vi "HFRR ADV v027 new software.vi"() -> ()   [LabVIEW 2025] (continued)
                      n2898 = Fract/Exp String To Number(string=w3966) -> (number=→"MWSD 2":dbl)  [unwired: 3 in, 1 out]
                    }
                    frame 11 {
                      n2899 = Fract/Exp String To Number(string=w3968) -> (number=→"AVP 2":dbl)  [unwired: 3 in, 1 out]
                    }
                    frame 12 {
                      n2900 = Fract/Exp String To Number(string=w3970) -> (number=→"HCF 2":dbl)  [unwired: 3 in, 1 out]
                    }
                    frame 13 {
                      n2901 = Fract/Exp String To Number(string=w3972) -> (number=→"WS1.4 2":dbl)  [unwired: 3 in, 1 out]
                    }
                    frame 14, Default {
                    }
                  }
                }
              }
              frame #2 {
              }
            }
            n2902 = local write "OK Button 16"(FALSE ("OK Button 13")) -> ()
          }
        }
        n2903 = Index Array(array=w3617, index="Select Printer 3") -> (element=w3619:string)
        "Selected Printer" <- w3619
        n2904 = case shown="True" w3614 {
          frame False {
          }
          frame True {
            n2905 = flat-sequence {
              frame #0 {
              }
              frame #1 {
                n2906 = Wait (ms)(milliseconds to wait=u32 100) -> ()  [unwired: 1 out]
              }
              frame #2 {
                n2907 = local write "OK Button 16"(FALSE ("Print 3")) -> ()
              }
            }
          }
        }
        n2908 = case shown="True" "Print" {
          tunnel: w3619 -> [_ w3911]
          frame False {
          }
          frame True {
            (unwired) i16 6 ("width (-)")
            (unwired) "TESTED BY : "
            (unwired) "TESTED DATE :"
            (unwired) "SAMPLE ID : "
            (unwired) "SAMPLE DESIGN : "
            w3869 = "\r"
            w3886 = "\r"
            # "add image"
            n2909 = local read "Sample ID"() -> (w3859:string)
            n2910 = local read "Tested by"() -> (w3862:string)
            n2911 = local read "String 34"() -> (w3849:string)
            n2912 = local read "String 45"() -> (w3829:string)
            n2913 = local read "String 35"() -> (w3844:string)
            n2914 = local read "String 37"() -> (w3842:string)
            n2915 = local read "String 32"() -> (w3864:string)
            n2916 = local read "String 36"() -> (w3839:string)
            n2917 = local read "String 31"() -> (w3863:string)
            n2918 = local read "Test Date"() -> (w3860:string)
            n2919 = local read "String 33"() -> (w3865:string)
            n2920 = local read "String 38"() -> (w3835:string)
            n2921 = local read "String 39"() -> (w3832:string)
            n2922 = local write "Print"(FALSE ("Print FF")) -> ()
            n2923 = local read "S 39"() -> (w3847:string)
            n2924 = local read "S 38"() -> (w3854:string)
            n2925 = local read "Temperature before test 2"() -> (w3885:dbl)
            n2926 = local read "Temperature after test 2"() -> (w3875:dbl)
            n2927 = local read "Humidity before test 2"() -> (w3900:dbl)
            n2928 = local read "Humidity after test 2"() -> (w3884:dbl)
            n2929 = local read "MWSD 2"() -> (w3889:dbl)
            n2930 = local read "WS1.4 2"() -> (w3867:dbl)
            n2931 = Concatenate Strings("2)" ("string"), w3849) -> (w3850:string)
            n2932 = Concatenate Strings("3)" ("string"), w3847) -> (w3848:string)
            n2933 = Concatenate Strings("1)" ("string"), w3854) -> (w3853:string)
            n2934 = Concatenate Strings("4)" ("string"), w3844) -> (w3845:string)
            n2935 = Concatenate Strings("5)" ("string"), w3842) -> (w3841:string)
            n2936 = Concatenate Strings("6)" ("string"), w3839) -> (w3838:string)
            n2937 = Concatenate Strings("7)" ("string"), w3835) -> (w3836:string)
            n2938 = Concatenate Strings("8)" ("string"), w3832) -> (w3833:string)
            n2939 = local read "HCF 2"() -> (w3871:dbl)
            n2940 = local read "AVP 2"() -> (w3888:dbl)
            n2941 = local read "s.NO"() -> (w3830:string)
            n2942 = call <vilib>:"New Report.vi"("report type"=enum16{"Standard Report", "HTML"}."Standard Report") -> ("report out"=w3909:refnum<class "NI_report.lvclass">, "error out"=w3908:errorcluster)  [unwired: 13 in]
            n2943 = local read "TITTLE"() -> (w3861:string)
            n2944 = Concatenate Strings(w3886, w3829, w3830, w3886, w3864, w3859, w3886, w3863, w3860, w3886, w3865, w3862, w3886) -> (w3879:string)
            "test by" <- w3879
            n2945 = Number To Fractional String(number=w3885, width (-)=i16 6, precision (6)=i16 2) -> (F-format string=w3874:string)  [unwired: 1 in]
            n2946 = Number To Fractional String(number=w3884, width (-)=i16 6, precision (6)=i16 2) -> (F-format string=w3887:string)  [unwired: 1 in]
            n2947 = Number To Fractional String(number=w3900, width (-)=i16 6, precision (6)=i16 2) -> (F-format string=w3905:string)  [unwired: 1 in]
            n2948 = Number To Fractional String(number=w3889, width (-)=i16 6, precision (6)=i16 2) -> (F-format string=w3891:string)  [unwired: 1 in]
            n2949 = Number To Fractional String(number=w3875, width (-)=i16 6, precision (6)=i16 2) -> (F-format string=w3876:string)  [unwired: 1 in]
            n2950 = Number To Fractional String(number=w3888, width (-)=i16 6, precision (6)=i16 2) -> (F-format string=w3890:string)  [unwired: 1 in]
            n2951 = Number To Fractional String(number=w3871, width (-)=i16 6, precision (6)=i16 2) -> (F-format string=w3870:string)  [unwired: 1 in]
            n2952 = Number To Fractional String(number=w3867, precision (6)=i16 2) -> (F-format string=w3866:string)  [unwired: 2 in]
            n2953 = call-dynamic "Set Report Header Text.vi"("report in"=w3909, "center header text"=w3861, "error in (no error)"=w3908) -> ("report out"=w3880:refnum<class "NI_report.lvclass">, "error out"=w3881:errorcluster)  [unwired: 11 in]
            n2954 = Concatenate Strings(w3869, w3853, w3905, w3869, w3850, w3874, w3869, w3848, w3887, w3869, w3845, w3876, w3869, w3841, w3891, w3869, w3838, w3890, w3869, w3836, w3870, w3869, w3833, w3866) -> (w3857:string)
            "export 2" <- w3857
            n2955 = call-poly <vilib>:"Append Report Text.vi"("report in"=w3880, "text"=w3879, "error in (no error)"=w3881) -> ("report out"=w3883:refnum<class "NI_report.lvclass">, "error out"=w3882:errorcluster)  [unwired: 9 in, 2 out]
            n2956 = local read "test by"() -> (w3856:string)
            n2957 = local read "TITTLE"() -> (w3858:string)
            n2958 = call-poly <vilib>:"Append Report Text.vi"("report in"=w3883, "error in (no error)"=w3882) -> ("report out"=w3904:refnum<class "NI_report.lvclass">, "error out"=w3902:errorcluster)  [unwired: 10 in, 2 out]
            n2959 = Concatenate Strings(w3858, w3857, w3856) -> (→"output":string)
            n2960 = call-poly <vilib>:"Append Report Text.vi"("report in"=w3904, "text"=w3857, "error in (no error)"=w3902) -> ("report out"=w3903:refnum<class "NI_report.lvclass">, "error out"=w3901:errorcluster)  [unwired: 9 in, 2 out]
            n2961 = call-dynamic "Print Report.vi"("report in"=w3903, "printer name (default)"=w3911, "error in (no error)"=w3901) -> ("report out"=w3913:refnum<class "NI_report.lvclass">, "error out"=w3914:errorcluster)  [unwired: 11 in]
            n2962 = call-dynamic "Dispose Report.vi"("report in"=w3913, "error in (no error)"=w3914) -> ()  [unwired: 13 in, 1 out]
          }
        }
        n2963 = case shown="True" "Print 2" {
          frame False {
          }
          frame True {
            n2964 = flat-sequence {
              frame #0 {
                n2965 = local read "s.NO"() -> (→"s.NO 2":string)
                n2966 = Wait (ms)(milliseconds to wait=u32 20) -> ()  [unwired: 1 out]
                n2967 = local read "Sample ID  3"() -> (→"Sample ID  6":string)
                n2968 = local read "Sample ID  4"() -> (→"Sample ID  7":string)
                n2969 = local read "Sample ID"() -> (→"Sample ID  2":string)
                n2970 = local read "Tested by"() -> (→"Tested by 2":string)
                n2971 = local read "Test Date"() -> (→"Test Date 2":string)
                n2972 = local read "Humidity after test 3"() -> (→"Humidity after test 4":dbl)
                n2973 = local read "Ref A Test Date :"() -> (→"TITTLE 4":string)
                n2974 = local read "Temperature before test 3"() -> (w3736:dbl)
                n2975 = local read "Temperature before test 3"() -> (→"Temperature after test 5":dbl)
                n2976 = local read "Temperature after test 3"() -> (→"Temperature after test 4":dbl)
                n2977 = local read "Humidity before test 3"() -> (→"Humidity before test 4":dbl)
                n2978 = local write "Temperature before test 3"(w3736) -> ()
                n2979 = local read "image data"() -> (w3727:T16)
                n2980 = String To Path(string="C:\\LAB-IQ\\im\\Temp_resized.jpg") -> (path=w3728:path)
                "path 2" <- w3728
                n2981 = call <vilib>:"Write JPEG File.vi"("image data"=w3727, "path to JPEG file"=w3728) -> ()  [unwired: 8 in, 2 out]
                "Ref A Test Date :" <- "Ref A Test Date :"
                "Ref B Test Date :" <- "Ref B Test Date :"
                "Ref B Scar Value :" <- "Ref B Scar Value :"
                "Ref A Scar Value :" <- "Ref A Scar Value :"
              }
              frame #1 {
                (unwired) HTML_Report_Image_Alignment."MIDDLE" ("alignment (default)")
                w3764 = u16 0 items=["portrait", "landscape"] ("orientation (portrait)")
                (unwired) HTML_Report_Image_Alignment."ABSMIDDLE" ("alignment (default)")
                (unwired) "TESTED BY : "
                (unwired) "TESTED DATE :"
                (unwired) "SAMPLE ID : "
                (unwired) "SAMPLE DESIGN : "
                w3797 = "\r"
                # "add image"
                n2982 = Wait (ms)(milliseconds to wait=u32 20) -> ()  [unwired: 1 out]
                n2983 = local read "Sample ID  2"() -> (w3790:string)
                n2984 = local read "Wear Scar X"() -> (w3762:dbl)
                "Length ( microns ) 2" <- w3762
                n2985 = local read "Wear Scar Y"() -> (w3761:dbl)
                "Wear Scar Y ( microns ) :" <- w3761
                n2986 = local read "Test Date 2"() -> (w3791:string)
                n2987 = local read "Tested by 2"() -> (w3792:string)
                n2988 = local read "String 46"() -> (w3788:string)
                n2989 = local read "String 48"() -> (w3794:string)
                n2990 = local read "String 47"() -> (w3793:string)
                n2991 = local read "String 49"() -> (w3795:string)
                n2992 = local read "String 10"() -> (w3748:string)
                n2993 = local read "s.NO 2"() -> (w3789:string)
                n2994 = Add(x=w3762, y=w3761) -> (x+y=w3760:dbl)
                n2995 = call <vilib>:"New Report.vi"("report type"=enum16{"Standard Report", "HTML"}."HTML") -> ("report out"=w3768:refnum<class "NI_report.lvclass">, "error out"=w3766:errorcluster)  [unwired: 13 in]
                n2996 = Concatenate Strings(w3797, w3788, w3789, w3797, w3794, w3790, w3797, w3793, w3791, w3797, w3795, w3792, w3797) -> (→"test by 2":string)
                n2997 = Concatenate Strings("C:\\LAB-IQ\\Data\\" ("string"), w3748, ".jpg" ("string")) -> ()  [unwired: 1 out]
                n2998 = Divide(x=w3760, y=2.0) -> (x/y=→"Mean Wear ( microns) :":dbl)
                n2999 = call-dynamic "Set Report Orientation.vi"("report in"=w3768, "orientation (portrait)"=w3764, "error in (no error)"=w3766) -> ("report out"=w3767:refnum<class "NI_report.lvclass">, "error out"=w3765:errorcluster)  [unwired: 11 in]
                n3000 = for {
                  N: 5 -> [_]
                  tunnel: w3767 -> [w3818]
                  tunnel: [w3817] -> w3746
                  tunnel: w3765 -> [w3816]
                  tunnel: [w3815] -> w3745
                  n3001 = call-dynamic "Set Report Tab Width.vi"("report in"=w3818, "error in (no error)"=w3816) -> ("report out"=w3817:refnum<class "NI_report.lvclass">, "error out"=w3815:errorcluster)  [unwired: 12 in]
                }
                n3002 = local read "TITTLE"() -> (w3763:string)
                n3003 = call-dynamic "Set Report Header Text.vi"("report in"=w3746, "center header text"=w3763, "error in (no error)"=w3745) -> ("report out"=w3784:refnum<class "NI_report.lvclass">, "error out"=w3783:errorcluster)  [unwired: 11 in]
                n3004 = for {
                  N: 1 -> [_]
                  tunnel: [w3822] -> w3770
                  tunnel: [w3821] -> w3769
                  tunnel: w3784 -> [w3820]
                  tunnel: w3783 -> [w3819]
                  n3005 = call-dynamic "New Report Line.vi"("report in"=w3820, "error in (no error)"=w3819) -> ("report out"=w3822:refnum<class "NI_report.lvclass">, "error out"=w3821:errorcluster)  [unwired: 12 in]
                }
                n3006 = for {
                  N: 2 -> [_]
                  tunnel: [w3814] -> w3776
                  tunnel: [w3813] -> w3775
                  tunnel: w3770 -> [w3812]
                  tunnel: w3769 -> [w3811]
                  n3007 = call-dynamic "New Report Line.vi"("report in"=w3812, "error in (no error)"=w3811) -> ("report out"=w3814:refnum<class "NI_report.lvclass">, "error out"=w3813:errorcluster)  [unwired: 12 in]
                }
                n3008 = for {
                  N: 25 -> [_]
                  tunnel: w3776 -> [w3810]
                  tunnel: w3775 -> [w3808]
                  tunnel: [w3809] -> w3779
                  tunnel: [w3807] -> w3778
                  n3009 = call-dynamic "Set Report Tab Width.vi"("report in"=w3810, "error in (no error)"=w3808) -> ("report out"=w3809:refnum<class "NI_report.lvclass">, "error out"=w3807:errorcluster)  [unwired: 12 in]
                }
                n3010 = control-ref of="Tab Control 9"() -> (w3774:refnum<vi>)
                n3011 = call-dynamic "Append Control Image to Report.vi"("report in"=w3779, "alignment (default)"=HTML_Report_Image_Alignment."ABSMIDDLE", "ctrl reference"=w3774, "error in (no error)"=w3778) -> ("report out"=w3773:refnum<class "NI_report.lvclass">, "error out"=w3772:errorcluster)  [unwired: 8 in, 2 out]
                n3012 = for {
                  N: 3 -> [_]
                  tunnel: [w3806] -> w3757
                  tunnel: [w3805] -> w3756
                  tunnel: w3773 -> [w3804]
                  tunnel: w3772 -> [w3803]
                  n3013 = call-dynamic "New Report Line.vi"("report in"=w3804, "error in (no error)"=w3803) -> ("report out"=w3806:refnum<class "NI_report.lvclass">, "error out"=w3805:errorcluster)  [unwired: 12 in]
                }
                n3014 = for {
                  N: 100 -> [_]
                  tunnel: w3757 -> [w3802]
                  tunnel: w3756 -> [w3800]
                  tunnel: [w3801] -> w3753
                  tunnel: [w3799] -> w3751
                  n3015 = call-dynamic "Set Report Tab Width.vi"("report in"=w3802, "error in (no error)"=w3800) -> ("report out"=w3801:refnum<class "NI_report.lvclass">, "error out"=w3799:errorcluster)  [unwired: 12 in]
                }
                n3016 = String To Path(string="C:\\LAB-IQ\\im\\Temp_resized.jpg") -> (path=w3743:path)
                n3017 = call-poly <vilib>:"Append Image to Report.vi"("report in"=w3753, "path or URL of image"=w3743, "error in (no error)"=w3751) -> ("report out"=w3752:refnum<class "NI_report.lvclass">, "error out"=w3750:errorcluster)  [unwired: 9 in, 2 out]
                n3018 = call-poly <vilib>:"Open HTML Report in Browser.vi"("report in"=w3752, "error in (no error)"=w3750) -> ("report out"=w3787:refnum<class "NI_report.lvclass">, "error out"=w3786:errorcluster)  [unwired: 11 in, 1 out]
                n3019 = call-dynamic "Dispose Report.vi"("report in"=w3787, "error in (no error)"=w3786) -> ()  [unwired: 13 in, 1 out]
              }
              frame #2 {
              }
              frame #3 {
                n3020 = disable-structure shown="Disabled" {
                  frame Disabled {
                    n3021 = local read "String 10"() -> (w3827:string)
                    n3022 = Concatenate Strings("C:\\LAB-IQ-NXT\\Data\\" ("string"), w3827, ".jpg" ("string")) -> (w3825:string)
                    n3023 = String To Path(string=w3825) -> (path=w3824:path)
                    n3024 = Delete(path (use dialog)=w3824) -> ()  [unwired: 4 in, 3 out]
                  }
                  frame Enabled {
                  }
                }
                n3025 = local write "Print 2"(FALSE ("Print")) -> ()
              }
            }
          }
        }
      }
    }
    n3026 = Wait (ms)(milliseconds to wait=u32 50) -> ()  [unwired: 1 out]
    n3027 = Wait (ms)(milliseconds to wait=u32 50) -> ()  [unwired: 1 out]
    n3028 = local read "Quit"() -> (w2172:bool)
  }
  n3029 = VISA Close(VISA resource name=w41, error in (no error)=w40) -> ()  [unwired: 1 out]
  n3030 = while {
    tunnel: [w3990] -> w49
    shift-right: [w3983] -> _
    shift-left: 0.0 -> [w3986]
    shift-right: [w3982] -> _
    shift-left: 0.0 -> [w3985]
    shift-right: [w3981] -> _
    shift-left: 100.0 ("vc_cmd") -> [w3984]
    stop <- w3990 stop-if-true
    # "PID LOGIC"
    n3031 = local read "run test Calibration"() -> (w3978:bool)
    n3032 = local read "RUN"() -> (w3988:bool)
    n3033 = local read "Auto Start Temp"() -> (w3979:bool)
    n3034 = local read "Auto Start Test"() -> (w3987:bool)
    n3035 = local read "START TEMP"() -> (w3977:bool)
    n3036 = And(x=w3979, y=w3987) -> (x .and. y?=w3980:bool)
    n3037 = Or(x=w3988, y=w3980) -> (x .or. y?=w3989:bool)
    n3038 = And(x=w3989, y=w3977) -> (x .and. y?=w3976:bool)
    n3039 = And(x=w3978, y=w3977) -> (x .and. y?=w3975:bool)
    n3040 = Or(x=w3975, y=w3976) -> (x .or. y?=w3974:bool)
    n3041 = Wait (ms)(milliseconds to wait="milliseconds to wait") -> ()  [unwired: 1 out]
    n3042 = case shown="True" w3974 {
      tunnel: [400.0 ("out_vc_cmd") w4009] -> w3981
      tunnel: [w3993 w4011] -> w3982
      tunnel: [w3993 w4010] -> w3983
      tunnel: w3986 -> [_ w4000]
      tunnel: w3985 -> [_ w3999]
      tunnel: w3984 -> [_ w3998]
      tunnel: w3978 -> [_ w3994]
      frame False {
        w3993 = 0.0 ("error_out")
      }
      frame True {
        n3043 = case shown="True" w3994 {
          tunnel: [w4018 1.0] -> w3996
          frame False {
            n3044 = local read "Set Strk"() -> (w4017:dbl)
            n3045 = Add(x=w4017, y="Add up Stroke") -> (x+y=w4018:dbl)
          }
          frame True {
          }
        }
        n3046 = local read "LVDT STROKE"() -> (w3995:dbl)
        n3047 = formula code="// Zero-Hardcode Explicit Positional-Form PID Engine\n// Inputs: target_stroke, measured_stroke, dt, prev_error, integral_accumulator_in, prev_vc_cmd\n//         kp, ki, kd, max_step_change, max_amplitude, min_amplitude, startup_cmd\n// Outputs: vc_cmd, error_out, out_error, integral_accumulator_out, out_vc_cmd\n\n// 1. Calculate Tracking Error\nfloat current_error = target_stroke - measured_stroke;\nerror_out = current_error;\n\n// 2. Compute Proportional Term\nfloat p_term = kp * current_error;\n\n// 3. Compute Derivative Term\nfloat d_term = 0.0;\nif (dt > 0.0) {\n    d_term = kd * ((current_error - prev_error) / dt);\n}\n\n// 4. Update and Accumulate Integral Term\nfloat current_integral = integral_accumulator_in + (current_error * dt);\nfloat i_term = ki * current_integral;\n\n// 5. Calculate Ideal Target Command\nfloat ideal_command = startup_cmd + p_term + i_term + d_term;\n\n// 6. Anti-Windup Protection (Back-calculation method)\nif (ideal_command > max_amplitude) {\n    float excess = ideal_command - max_amplitude;\n    if (ki > 0.0) {\n        current_integral -= excess / ki;\n    }\n    ideal_command = max_amplitude;\n} else if (ideal_command < min_amplitude) {\n    float excess = ideal_command - min_amplitude;\n    if (ki > 0.0) {\n        current_integral -= excess / ki;\n    }\n    ideal_command = min_amplitude;\n}\n\n// 7. Apply Loop Rate Limiting (Protects voice coil from large voltage steps)\nfloat raw_adjustment = ideal_command - prev_vc_cmd;\n\nif (raw_adjustment > max_step_change) {\n    raw_adjustment = max_step_change;\n} else if (raw_adjustment < -max_step_change) {\n    raw_adjustment = -max_step_change;\n}\n\nfloat next_vc_cmd = prev_vc_cmd + raw_adjustment;\n\n// Final Output Safety Safeguard Clamping\nif (next_vc_cmd > max_amplitude) {\n    next_vc_cmd = max_amplitude;\n} else if (next_vc_cmd < min_amplitude) {\n    next_vc_cmd = min_amplitude;\n}\n\n// 8. Map to Shift Registers for memory persistence\nvc_cmd = next_vc_cmd;\nout_error = current_error;                     \nintegral_accumulator_out = current_integral;  \nout_vc_cmd = next_vc_cmd;"("target_stroke"=w3996, "measured_stroke"=w3995, "dt"="dt", "integral_accumulator_in"=w3999, "prev_error"=w4000, "prev_vc_cmd"=w3998, "kp"="kp", "ki"="ki", "kd"="kd", "max_step_change"="max_step_change", "max_amplitude"="max_amplitude", "min_amplitude"="min_amplitude", "startup_cmd"="startup_cmd") -> ("vc_cmd"=w4015:dbl, "out_error"=w4010:dbl, "integral_accumulator_out"=w4011:dbl, "out_vc_cmd"=w4009:dbl)  [unwired: 1 out]
        "output Vpp" <- w4015
        n3048 = Number To Fractional String(number=w4015, precision (6)=i16 1) -> (F-format string=w4013:string)  [unwired: 2 in]
        n3049 = Concatenate Strings("DAC;" ("string"), w4013) -> (w3997:string)
        n3050 = local write "Due Write"(w3997) -> ()
        "prev_error" <- w4000
        "integral_accumulator_in" <- w3999
        "prev_vc_cmd" <- w3998
      }
    }
    n3051 = local read "Quit"() -> (w3990:bool)
  }
  n3052 = Or(x=w45, y=w44) -> (x .or. y?=w46:bool)
  n3053 = Or(x=w42, y=w46) -> (x .or. y?=w51:bool)
  n3054 = control-ref of="new picture"() -> ()  [unwired: 1 out]
  n3055 = Or(x=w54, y=w51) -> (x .or. y?=w48:bool)
  n3056 = Or(x=w48, y=w49) -> (x .or. y?=w43:bool)
  n3057 = while {
    tunnel: [w4020] -> w53
    i -> [w4027]
    stop <- w4020 stop-if-true
    n3058 = local read "Quit"() -> (w4020:bool)
    n3059 = Equal To 0?(x=w4027) -> (x = 0?=w4025:bool)
    n3060 = call "Elapsed Time3"("Time Target (s)"=45.0, "Auto Reset"=TRUE) -> ("Time has Elapsed"=w4024:bool)  [unwired: 10 in, 7 out]
    n3061 = Wait (ms)(milliseconds to wait=u32 50) -> ()  [unwired: 1 out]
    n3062 = Or(x=w4024, y=w4025) -> (x .or. y?=w4026:bool)
    n3063 = case shown="True" w4026 {
      frame False {
      }
      frame True {
        n3064 = call <vilib>:"System Exec.vi"("run minimized? (F)"=TRUE, "error in (no error)"="error in (no error)", "command line"="powercfg.exe -change -monitor-timeout-ac 0") -> ("error out"=w4038:errorcluster)  [unwired: 5 in, 3 out]
        n3065 = call <vilib>:"System Exec.vi"("run minimized? (F)"=TRUE, "error in (no error)"=w4038, "command line"="powercfg.exe -change -disk-timeout-ac 0") -> ("error out"=w4037:errorcluster)  [unwired: 5 in, 3 out]
        n3066 = call <vilib>:"System Exec.vi"("run minimized? (F)"=TRUE, "error in (no error)"=w4037, "command line"="powercfg.exe -change -standby-timeout-ac 0") -> ("error out"=w4036:errorcluster)  [unwired: 5 in, 3 out]
        n3067 = call <vilib>:"System Exec.vi"("run minimized? (F)"=TRUE, "error in (no error)"=w4036, "command line"="powercfg.exe -change -hibernate-timeout-ac 0") -> ("error out"=w4035:errorcluster)  [unwired: 5 in, 3 out]
        n3068 = call <vilib>:"Simple Error Handler.vi"("error in (no error)"=w4035) -> ("error out"=w4041:errorcluster)  [unwired: 4 in, 4 out]
        n3069 = call <vilib>:"Clear Errors.vi"("error in (no error)"=w4041) -> ("error out"=→"error out":errorcluster)  [unwired: 5 in, 1 out]
      }
    }
  }
  n3070 = Compound Arithmetic op=OR(w56, w43, w53) -> (w55:bool)
  n3071 = flat-sequence {
    tunnel: w55 -> [_]
    tunnel: [w4043] -> w25
    tunnel: w25 -> [_]
    frame #0 {
      n3072 = call "CLOSE CONNECTION.vi"() -> ("error out"=w4043:errorcluster)  [unwired: 11 in]
    }
    frame #1 {
      n3073 = Quit LabVIEW(quit? (T)=TRUE) -> ()
      n3074 = local write "Quit"(FALSE ("EXIT")) -> ()
    }
  }
  n3075 = property on="Heater Button" class="Bool (strict)"("Visible"=TRUE) -> ()  [unwired: 2 in, 2 out]
  n3076 = while {
    tunnel: [w4050] -> _
    i -> [w4050]
    stop <- w4046 stop-if-true
    # "Langauage selection"
    n3077 = Equal?(x="Lan flag", y=22.0) -> ()  [unwired: 1 out]
    n3078 = disable-structure shown="Disabled" {
      frame Disabled {
        n3079 = stacked-sequence {
          frame #0 {
            n3080 = case shown="\"Russian\"" "Language Selection" {
              tunnel: [0 1] -> w4052
              frame "English", Default {
              }
              frame "Russian" {
              }
            }
            n3081 = for {
              N: 130 -> [_]
              tunnel: "Table" -> [w4061]
              tunnel: w4052 -> [w4060]
              i -> [w4059]
              n3082 = Index Array(array=w4061, index (row)=w4059, index (col)=w4060) -> (element=w4058:string)
              n3083 = case shown="1" w4059 {
                tunnel: w4058 -> [w4062 w4063 _ w4064 w4065 w4066 w4067 w4068 w4069 w4070 w4071 w4072 w4073 w4074 w4075 w4076 w4077 w4078 w4079 w4080 w4081 w4082 w4083 w4084 w4085 w4086 w4087 w4088 w4089 _ _ w4090 w4091 w4092 w4093 w4094 w4095 w4104 w4111 w4118 w4125 w4129 w4132 w4135 w4137 w4139 w4140 w4141 w4142 w4143 w4144 w4145 w4146 w4147 w4148 w4149 w4150 w4151 w4152 w4153 w4154 w4155 w4156 w4157 w4158 w4159 w4160 w4161 w4162 w4163 w4164 w4165 w4166 w4167 w4168 w4169 w4170 w4171 w4172 w4173 w4174 w4175 w4176 w4177 w4178 w4179 w4180 w4181 w4182 w4183 w4184 w4185 w4186 w4187 w4188 w4189 w4190 w4191 w4192 w4193 w4194 w4195 w4196 w4197 w4198 _ w4199 w4200 w4201 w4202 w4203 w4204 w4205 w4206 w4207 w4208 w4209 w4210 w4211 _ w4212 w4213 w4214 w4215 w4216 w4217 _]
                frame 0 {
                  n3084 = local write "S"(w4062) -> ()
                }
                frame 1 {
                  n3085 = local write "S 2"(w4063) -> ()
                }
                frame 2 {
                }
                frame 3 {
                  n3086 = local write "S 4"(w4064) -> ()
                }
                frame 4 {
                  n3087 = property on="FILE" class="Str"("Caption.Text"=w4065) -> ()  [unwired: 2 in, 2 out]
                }
                frame 5 {
                  n3088 = property on="Fuel Discription :" class="Str"("Caption.Text"=w4066) -> ()  [unwired: 2 in, 2 out]
                }
                frame 6 {
                  n3089 = property on="Remarks :" class="Str"("Caption.Text"=w4067) -> ()  [unwired: 2 in, 2 out]
                }
                frame 7 {
                  n3090 = property on="Save & Continue" class="Bool (strict)"("Boolean Text.Text"=w4068) -> ()  [unwired: 2 in, 2 out]
                }
                frame 8 {
                }
                frame 9 {
                  n3091 = property on="Set Hz" class="DigNum (strict)"("Caption.Text"=w4070) -> ()  [unwired: 2 in, 2 out]
                }
                frame 10 {
                }
                frame 11 {
                  n3092 = property on="NORMAL LOAD" class="DigNum (strict)"("Caption.Text"=w4072) -> ()  [unwired: 2 in, 2 out]
                }
                frame 12 {
                }
                frame 13 {
                  n3093 = property on="Set Temp" class="DigNum (strict)"("Caption.Text"=w4074) -> ()  [unwired: 2 in, 2 out]
                }
                frame 14 {
                  n3094 = local write "S 15"(w4075) -> ()
                }
                frame 15 {
                  n3095 = property on="Set Rh" class="DigNum (strict)"("Caption.Text"=w4076) -> ()  [unwired: 2 in, 2 out]
                }
                frame 16 {
                }
                frame 17 {
                  n3096 = local write "S 18"(w4078) -> ()
                }
                frame 18 {
                  "String 17" <- w4079
                }
                frame 19 {
                  n3097 = property on="test time" class="DigNum (strict)"("Caption.Text"=w4080) -> ()  [unwired: 2 in, 2 out]
                }
                frame 20 {
                  "String 18" <- w4081
                  "String 22" <- w4081
                }
                frame 21 {
                  n3098 = property on="Elapsed time" class="DigNum (strict)"("Caption.Text"=w4082) -> ()  [unwired: 2 in, 2 out]
                }
                frame 22 {
                  n3099 = property on="Samplingtime 2" class="DigNum (strict)"("Caption.Text"=w4083) -> ()  [unwired: 2 in, 2 out]
                }
                frame 23 {
                  "String 21" <- w4084
                }
                frame 24 {
                  n3100 = property on="Countdown" class="DigNum (strict)"("Caption.Text"=w4085) -> ()  [unwired: 2 in, 2 out]
                }
                frame 25 {
                  n3101 = property on="Countdown 2" class="DigNum (strict)"("Caption.Text"=w4086) -> ()  [unwired: 2 in, 2 out]
                }
                frame 26 {
                  n3102 = property on="Engage" class="Bool (strict)"("Boolean Text.Text"=w4087) -> ()  [unwired: 2 in, 2 out]
                }
                frame 27 {
                  n3103 = property on="Boolean  4" class="Bool (strict)"("Boolean Text.Text"=w4088) -> ()  [unwired: 2 in, 2 out]
                }
                frame 28 {
                  n3104 = property on="Test \nStatus" class="Bool (strict)"("Boolean Text.Text"=w4089) -> ()  [unwired: 2 in, 2 out]
                }
                frame 29 {
                }
                frame 30 {
                }
                frame 31 {
                }
                frame 32 {
                  n3105 = property on="RSTCOF" class="Bool"("Boolean Text.Text"=w4091) -> ()  [unwired: 2 in, 2 out]
                  n3106 = property on="RST FF" class="Bool"("Boolean Text.Text"=w4091) -> ()  [unwired: 2 in, 2 out]
                  n3107 = property on="RST TEMP" class="Bool"("Boolean Text.Text"=w4091) -> ()  [unwired: 2 in, 2 out]
                  n3108 = property on="RSTV1 3" class="Bool"("Boolean Text.Text"=w4091) -> ()  [unwired: 2 in, 2 out]
                  n3109 = property on="rstv2" class="Bool"("Boolean Text.Text"=w4091) -> ()  [unwired: 2 in, 2 out]
                  n3110 = property on="RSTV1 2" class="Bool"("Boolean Text.Text"=w4091) -> ()  [unwired: 2 in, 2 out]
                  n3111 = property on="RST CP" class="Bool"("Boolean Text.Text"=w4091) -> ()  [unwired: 2 in, 2 out]
                }
                frame 33 {
                  "S 61" <- w4092
                }
                frame 34 {
                  "String 23" <- w4093
                }
                frame 35 {
                  n3112 = property on="Rh Before" class="DigNum (strict)"("Caption.Text"=w4094) -> ()  [unwired: 2 in, 2 out]
                }
                frame 36 {
                  n3113 = Match Pattern(string=w4095, regular expression=",") -> (before substring=→"bs":string, after substring=→"as":string)  [unwired: 1 in, 2 out]
                  n3114 = property on="Rh After" class="DigNum (strict)"("Caption.Text"=w4095) -> ()  [unwired: 2 in, 2 out]
                }
                frame 37 {
                  n3115 = Match Pattern(string=w4104, regular expression=",") -> (before substring=w4103:string, after substring=w4102:string)  [unwired: 1 in, 2 out]
                  "bs" <- w4103
                  "as" <- w4102
                  n3116 = Concatenate Strings(w4103, w4102) -> (w4099:string)
                  n3117 = property on="Humidity before test 2" class="DigNum (strict)"("Caption.Text"=w4099) -> ()  [unwired: 2 in, 2 out]
                  n3118 = Concatenate Strings(w4099, "=" ("string")) -> (w4100:string)
                  n3119 = local write "S 38"(w4100) -> ()
                }
                frame 38 {
                  n3120 = Match Pattern(string=w4111, regular expression=",") -> (before substring=w4110:string, after substring=w4109:string)  [unwired: 1 in, 2 out]
                  "bs" <- w4110
                  "as" <- w4109
                  n3121 = Concatenate Strings(w4110, w4109) -> (w4106:string)
                  n3122 = property on="Humidity after test 2" class="DigNum (strict)"("Caption.Text"=w4106) -> ()  [unwired: 2 in, 2 out]
                  n3123 = Concatenate Strings(w4106, "=" ("string")) -> (w4108:string)
                  n3124 = local write "S 39"(w4108) -> ()
                }
                frame 39 {
                  n3125 = Match Pattern(string=w4118, regular expression=",") -> (before substring=w4117:string, after substring=w4116:string)  [unwired: 1 in, 2 out]
                  "bs" <- w4117
                  "as" <- w4116
                  n3126 = Concatenate Strings(w4117, w4116) -> (w4113:string)
                  n3127 = property on="Temperature before test 2" class="DigNum (strict)"("Caption.Text"=w4113) -> ()  [unwired: 2 in, 2 out]
                  n3128 = Concatenate Strings(w4113, "=" ("string")) -> (→"String 34":string)
                }
                frame 40 {
                  n3129 = Match Pattern(string=w4125, regular expression=",") -> (before substring=w4124:string, after substring=w4123:string)  [unwired: 1 in, 2 out]
                  "bs" <- w4124
                  "as" <- w4123
                  n3130 = Concatenate Strings(w4124, w4123) -> (w4120:string)
                  n3131 = property on="Temperature after test 2" class="DigNum (strict)"("Caption.Text"=w4120) -> ()  [unwired: 2 in, 2 out]
                  n3132 = Concatenate Strings(w4120, "=" ("string")) -> (→"String 35":string)
                  n3133 = property on="Temperature after test" class="DigNum (strict)"("Caption.Text"=w4120) -> ()  [unwired: 2 in, 2 out]
                }
                frame 41 {
                  n3134 = property on="AVP 2" class="DigNum (strict)"("Caption.Text"=w4129) -> ()  [unwired: 2 in, 2 out]
                  n3135 = Concatenate Strings(w4129, "=" ("string")) -> (→"String 36":string)
                }
                frame 42 {
                  n3136 = property on="MWSD 2" class="DigNum (strict)"("Caption.Text"=w4132) -> ()  [unwired: 2 in, 2 out]
                  n3137 = Concatenate Strings(w4132, "=" ("string")) -> (→"String 37":string)
                }
                frame 43 {
                  n3138 = property on="HCF 2" class="DigNum (strict)"("Caption.Text"=w4135) -> ()  [unwired: 2 in, 2 out]
                  n3139 = Concatenate Strings(w4135, "=" ("string")) -> (→"String 38":string)
                }
                frame 44 {
                  n3140 = Concatenate Strings(w4137, "=" ("string")) -> (→"String 39":string)
                  n3141 = property on="WS1.4 2" class="DigNum (strict)"("Caption.Text"=w4137) -> ()  [unwired: 2 in, 2 out]
                }
                frame 45 {
                }
                frame 46 {
                  n3142 = local write "S 47"(w4140) -> ()
                }
                frame 47 {
                  n3143 = local write "S 48"(w4141) -> ()
                }
                frame 48 {
                  n3144 = local write "S 49"(w4142) -> ()
                }
                frame 49 {
                  n3145 = local write "S 50"(w4143) -> ()
                }
                frame 50 {
                  n3146 = local write "S 51"(w4144) -> ()
                }
                frame 51 {
                  n3147 = local write "S 52"(w4145) -> ()
                }
                frame 52 {
                  n3148 = local write "S 53"(w4146) -> ()
                }
                frame 53 {
                  n3149 = local write "S 54"(w4147) -> ()
                }
                frame 54 {
                  n3150 = local write "S 55"(w4148) -> ()
                }
                frame 55 {
                  n3151 = local write "S 56"(w4149) -> ()
                }
                frame 56 {
                  n3152 = local write "S 57"(w4150) -> ()
                }
                frame 57 {
                  n3153 = local write "S 58"(w4151) -> ()
                }
                frame 58 {
                  n3154 = local write "S 59"(w4152) -> ()
                }
                frame 59 {
                  n3155 = local write "S 60"(w4153) -> ()
                }
                frame 60 {
                  n3156 = local write "S 62"(w4154) -> ()
                }
                frame 61 {
                  n3157 = local write "S 63"(w4155) -> ()
                }
                frame 62 {
                  n3158 = local write "S 64"(w4156) -> ()
                }
                frame 63 {
                  n3159 = local write "S 65"(w4157) -> ()
                }
                frame 64 {
                  n3160 = local write "S 66"(w4158) -> ()
                }
                frame 65 {
                  n3161 = local write "S 67"(w4159) -> ()
                }
                frame 66 {
                  n3162 = local write "S 68"(w4160) -> ()
                }
                frame 67 {
                  n3163 = local write "S 69"(w4161) -> ()
                }
                frame 68 {
                  n3164 = local write "S 70"(w4162) -> ()
                }
                frame 69 {
                  n3165 = local write "S 71"(w4163) -> ()
                }
                frame 70 {
                  n3166 = local write "S 72"(w4164) -> ()
                }
                frame 71 {
                  n3167 = local write "S 73"(w4165) -> ()
                }
                frame 72 {
                  n3168 = local write "S 74"(w4166) -> ()
                }
                frame 73 {
                  n3169 = local write "S 75"(w4167) -> ()
                }
                frame 74 {
                  n3170 = local write "S 76"(w4168) -> ()
                }
                frame 75 {
                  n3171 = local write "S 77"(w4169) -> ()
                }
                frame 76 {
                  n3172 = local write "S 78"(w4170) -> ()
                }
                frame 77 {
                  n3173 = local write "S 79"(w4171) -> ()
                }
                frame 79 {
                  n3174 = property on="Sample Temperature ( °C )" class="XYGraph (strict)"("Y Scale.Name Label.Text"=w4172) -> ()  [unwired: 2 in, 2 out]
                }
                frame 80 {
                  n3175 = local write "S 81"(w4173) -> ()
                  n3176 = property on="Humidity ( %RH )" class="XYGraph (strict)"("Y Scale.Name Label.Text"=w4173) -> ()  [unwired: 2 in, 2 out]
                }
                frame 78 {
                  n3177 = property on="Air Temperature  ( °C )" class="XYGraph (strict)"("X Scale.Name Label.Text"=w4174) -> ()  [unwired: 2 in, 2 out]
                  n3178 = property on="Humidity ( %RH )" class="XYGraph (strict)"("X Scale.Name Label.Text"=w4174) -> ()  [unwired: 2 in, 2 out]
                  n3179 = property on="Sample Temperature ( °C )" class="XYGraph (strict)"("X Scale.Name Label.Text"=w4174) -> ()  [unwired: 2 in, 2 out]
                  n3180 = property on="Coefficient Of Friction" class="XYGraph (strict)"("X Scale.Name Label.Text"=w4174) -> ()  [unwired: 2 in, 2 out]
                }
                frame 81 {
                  n3181 = property on="Air Temperature  ( °C )" class="XYGraph (strict)"("Y Scale.Name Label.Text"=w4175) -> ()  [unwired: 2 in, 2 out]
                }
                frame 82 {
                  n3182 = local write "S 84"(w4176) -> ()
                }
                frame 83 {
                  n3183 = local write "S 85"(w4177) -> ()
                }
                frame 84 {
                  n3184 = local write "S 86"(w4178) -> ()
                }
                frame 85 {
                  n3185 = local write "S 87"(w4179) -> ()
                }
                frame 86 {
                  n3186 = local write "S 88"(w4180) -> ()
                }
                frame 87 {
                }
                frame 88 {
                  n3187 = local write "S 90"(w4182) -> ()
                }
                frame 89 {
                  n3188 = local write "S 91"(w4183) -> ()
                }
                frame 90 {
                  n3189 = local write "S 92"(w4184) -> ()
                }
                frame 91 {
                  n3190 = local write "S 93"(w4185) -> ()
                }
                frame 92 {
                  n3191 = local write "S 94"(w4186) -> ()
                }
                frame 93 {
                  n3192 = local write "S 95"(w4187) -> ()
                }
                frame 94 {
                  n3193 = local write "S 96"(w4188) -> ()
                }
                frame 95 {
                  n3194 = local write "S 97"(w4189) -> ()
                }
                frame 96 {
                  n3195 = local write "S 98"(w4190) -> ()
                }
                frame 97 {
                  n3196 = local write "S 99"(w4191) -> ()
                }
                frame 98 {
                  n3197 = local write "S 100"(w4192) -> ()
                }
                frame 99 {
                  n3198 = local write "S 101"(w4193) -> ()
                }
                frame 100 {
                  n3199 = local write "S 102"(w4194) -> ()
                }
                frame 101 {
                  n3200 = local write "S 103"(w4195) -> ()
                }
                frame 102 {
                  n3201 = local write "S 104"(w4196) -> ()
                }
                frame 103 {
                  n3202 = local write "S 105"(w4197) -> ()
                }
                frame 104 {
                  n3203 = local write "S 106"(w4198) -> ()
                }
                frame 105 {
                }
                frame 106 {
                  n3204 = property on="OK Button 17" class="Bool (strict)"("Boolean Text.Text"=w4199) -> ()  [unwired: 2 in, 2 out]
                }
                frame 107 {
                  n3205 = property on="OK Button 16" class="Bool (strict)"("Boolean Text.Text"=w4200) -> ()  [unwired: 2 in, 2 out]
                }
                frame 108 {
                  n3206 = property on="TITTLE" class="Str"("Caption.Text"=w4201) -> ()  [unwired: 2 in, 2 out]
                }
                frame 109 {
                  "String 30" <- w4202
                }
                frame 110 {
                  n3207 = property on="Test Date" class="Str"("Caption.Text"=w4203) -> ()  [unwired: 2 in, 2 out]
                  "String 31" <- w4203
                }
                frame 111 {
                  n3208 = property on="Sample ID" class="Str"("Caption.Text"=w4204) -> ()  [unwired: 2 in, 2 out]
                  "String 32" <- w4204
                }
                frame 112 {
                  n3209 = property on="Tested by" class="Str"("Caption.Text"=w4205) -> ()  [unwired: 2 in, 2 out]
                  "String 33" <- w4205
                }
                frame 113 {
                  n3210 = property on="System Configured Printers 2" class="Arr (strict)"("Caption.Text"=w4206) -> ()  [unwired: 2 in, 2 out]
                }
                frame 114 {
                  n3211 = property on="Selected Printer" class="Str"("Caption.Text"=w4207) -> ()  [unwired: 2 in, 2 out]
                }
                frame 115 {
                  n3212 = property on="Select Printer 3" class="DigNum (strict)"("Caption.Text"=w4208) -> ()  [unwired: 2 in, 2 out]
                }
                frame 116 {
                  n3213 = property on="Print" class="Bool (strict)"("Boolean Text.Text"=w4209) -> ()  [unwired: 2 in, 2 out]
                }
                frame 117 {
                  "String 41" <- w4210
                }
                frame 118 {
                  n3214 = property on="tested by" class="Str"("Caption.Text"=w4211) -> ()  [unwired: 2 in, 2 out]
                }
                frame 119 {
                }
                frame 120 {
                  n3215 = property on="Export" class="Bool (strict)"("Boolean Text.Text"=w4212) -> ()  [unwired: 2 in, 2 out]
                }
                frame 121 {
                }
                frame 122 {
                }
                frame 123 {
                  n3216 = property on="Select File Type" class="Enum (strict)"("Caption.Text"=w4215) -> ()  [unwired: 2 in, 2 out]
                }
                frame 124 {
                  n3217 = property on="s.NO" class="Str"("Caption.Text"=w4216) -> ()  [unwired: 2 in, 2 out]
                  "String 45" <- w4216
                }
                frame 125 {
                  n3218 = property on="trip1 8" class="Bool (strict)"("Boolean Text.Text"=w4217) -> ()  [unwired: 2 in, 2 out]
                }
                frame 126, Default {
                }
              }
            }
          }
          frame #1 {
            w4225 = TRUE ("Visible")
            n3219 = local read "S 91"() -> (w4242:string)
            n3220 = local read "S 90"() -> (w4241:string)
            n3221 = local read "S 88"() -> (w4240:string)
            n3222 = property on="File Path" class="Path"("Caption.Text"=w4241) -> ()  [unwired: 2 in, 2 out]
            n3223 = local read "S 71"() -> (w4235:string)
            n3224 = local read "S 86"() -> (w4237:string)
            n3225 = local read "S 85"() -> (w4238:string)
            n3226 = local read "S 87"() -> (w4236:string)
            n3227 = local read "S 84"() -> (w4239:string)
            n3228 = local read "S 103"() -> (w4224:string)
            n3229 = local read "S 104"() -> (w4223:string)
            n3230 = property on="Password" class="Str"("Caption.Text"=w4238) -> ()  [unwired: 2 in, 2 out]
            n3231 = property on="EDIT" class="Bool (strict)"("Boolean Text.Text"=w4235) -> ()  [unwired: 2 in, 2 out]
            n3232 = property on="SAVE" class="Bool (strict)"("Boolean Text.Text"=w4239) -> ()  [unwired: 2 in, 2 out]
            n3233 = Build Array(w4224, w4223) -> (w4222:string[])
            n3234 = property on="Heater Button" class="Bool (strict)"("Strings [4]"=w4222) -> ()  [unwired: 2 in, 2 out]
            n3235 = local read "S 92"() -> (w4234:string)
            n3236 = local read "S 93"() -> (w4233:string)
            n3237 = local read "S 105"() -> (w4220:string)
            n3238 = local read "S 106"() -> (w4219:string)
            n3239 = Build Array(w4234, w4233) -> ()  [unwired: 1 out]
            n3240 = Build Array(w4220, w4219) -> (w4221:string[])
            n3241 = local read "S 95"() -> (w4231:string)
            n3242 = local read "S 94"() -> (w4232:string)
            n3243 = local read "bs"() -> (w4247:string)
            n3244 = local read "as"() -> (w4248:string)
            n3245 = property on="Humidity" class="Bool (strict)"("Strings [4]"=w4221) -> ()  [unwired: 2 in, 2 out]
            n3246 = Concatenate Strings(w4247, "\r", w4248) -> ()  [unwired: 1 out]
            n3247 = property on="Rh After" class="DigNum (strict)"("Caption.Size to Text?"=TRUE ("Caption.Size to Text")) -> ()  [unwired: 2 in, 2 out]
            n3248 = local read "S 48"() -> (w4271:string)
            n3249 = local read "S 50"() -> (w4269:string)
            n3250 = local read "S 51"() -> (w4268:string)
            n3251 = local read "S 49"() -> (w4270:string)
            n3252 = local read "S 52"() -> (w4267:string)
            n3253 = local read "as"() -> (w4252:string)
            n3254 = local read "bs"() -> (w4253:string)
            n3255 = local read "S 56"() -> (w4266:string)
            n3256 = local read "S 57"() -> (w4265:string)
            n3257 = local read "S 58"() -> (w4264:string)
            n3258 = local read "S 59"() -> (w4263:string)
            n3259 = property on="OPEN" class="Bool (strict)"("Boolean Text.Text"=w4267) -> ()  [unwired: 2 in, 2 out]
            n3260 = property on="OPEN 1" class="Bool (strict)"("Boolean Text.Text"=w4271) -> ()  [unwired: 2 in, 2 out]
            n3261 = property on="OPEN 2" class="Bool (strict)"("Boolean Text.Text"=w4270) -> ()  [unwired: 2 in, 2 out]
            n3262 = property on="OPEN 3" class="Bool (strict)"("Boolean Text.Text"=w4269) -> ()  [unwired: 2 in, 2 out]
            n3263 = property on="OPEN 4" class="Bool (strict)"("Boolean Text.Text"=w4268) -> ()  [unwired: 2 in, 2 out]
            n3264 = Concatenate Strings(w4253, "\r", w4252) -> ()  [unwired: 1 out]
            n3265 = local read "S 102"() -> (w4226:string)
            n3266 = property on="КОФ1" class="DigNum (strict)"("Caption.Text"=w4266) -> ()  [unwired: 2 in, 2 out]
            n3267 = local read "S 98"() -> (w4230:string)
            n3268 = local read "S 99"() -> (w4229:string)
            n3269 = local read "S 100"() -> (w4228:string)
            n3270 = local read "S 101"() -> (w4227:string)
            n3271 = property on="КОФ2" class="DigNum (strict)"("Caption.Text"=w4265) -> ()  [unwired: 2 in, 2 out]
            n3272 = property on="КОФ3" class="DigNum (strict)"("Caption.Text"=w4264) -> ()  [unwired: 2 in, 2 out]
            n3273 = property on="КОФ4" class="DigNum (strict)"("Caption.Text"=w4263) -> ()  [unwired: 2 in, 2 out]
            n3274 = local read "bs"() -> (w4251:string)
            n3275 = local read "as"() -> (w4250:string)
            n3276 = local read "S 60"() -> (w4262:string)
            n3277 = local read "S 54"() -> (w4272:string)
            n3278 = Concatenate Strings(w4251, "\r", w4250) -> ()  [unwired: 1 out]
            n3279 = Concatenate Strings(w4272, w4262) -> ()  [unwired: 1 out]
            n3280 = local read "S 77"() -> (→"String 43":string)
            n3281 = local read "S 76"() -> (w4245:string)
            n3282 = local read "S 78"() -> (w4244:string)
            n3283 = local read "S 71"() -> (w4256:string)
            n3284 = local read "S 66"() -> (w4261:string)
            n3285 = local read "S 67"() -> (w4260:string)
            n3286 = local read "S 68"() -> (w4259:string)
            n3287 = local read "S 69"() -> (w4258:string)
            n3288 = local read "S 70"() -> (w4257:string)
            n3289 = property on="AIR TEMP" class="DigNum (strict)"("Caption.Text"=w4244) -> ()  [unwired: 2 in, 2 out]
            n3290 = property on="Set Strk" class="DigNum (strict)"("Caption.Text"=w4245) -> ()  [unwired: 2 in, 2 out]
            n3291 = property on="SPEED OUT:" class="DigNum (strict)"("Caption.Text"=w4259) -> ()  [unwired: 2 in, 2 out]
            n3292 = property on="EDIT" class="Bool (strict)"("Boolean Text.Text"=w4256) -> ()  [unwired: 2 in, 2 out]
            n3293 = local read "S 79"() -> (w4243:string)
          }
          frame #2 {
          }
        }
        n3294 = local write "Lan flag"(10.0 ("Lan flag")) -> ()
      }
      frame Enabled {
      }
    }
    n3295 = Wait (ms)(milliseconds to wait=u32 2000) -> ()  [unwired: 1 out]
    n3296 = local read "Quit"() -> (w4046:bool)
  }
  n3297 = while {
    shift-right: [w4278] -> _
    shift-left: _ -> [w4279]
    shift-right: [w4276] -> _
    shift-left: T18 {"Read Heave and Surge"="", "Bytes at Heave Port"=0.0, "Heave and Surge COM Port:"="COM9", "Com Port 2"="COM7", "Residual Due"="", "Heave COM Status 2"=TRUE, "Heave COM Status"=TRUE, "Port 2"=TRUE, "Sway PPR"=6400.0, "Surge PPR"=6400.0, "Heave PPR"=6400.0, "Sway Pitch"=2.0, "Surge Pitch"=3.0, "Heave Pitch"=4.0, "Sway Pulses/mm"=320.0, "Surge Pulses/mm"=1600.0, "Heave Pulses/mm"=1600.0, "inner loop"=0.0, "Read Heave and Surge 2"="", "String 36"="", "Write S"=FALSE, "WriteCC1"=[""], "Heave COM Loop"=0, "LastCom"="", "EXIT"=FALSE, "Error Heave"={"status"=TRUE, "code"=-1073807343, "source"=""}} -> [w4275]
    shift-right: [w4273] -> _
    shift-left: enum16{"init", "MAIN", "Panel Close"}."init" -> [w4274]
    stop <- w4277 stop-if-true
    # "HUMIDITY LOOP LOGIC"
    n3298 = case shown="\"MAIN\"" w4274 {
      tunnel: w4279 -> [w4293 w4311 w4367 w4369]
      tunnel: [w4288 w4315 w4367 w4369] -> w4278
      tunnel: [_ _ TRUE _] -> w4277
      tunnel: [w4285 w4313 w4365 w4368] -> w4276
      tunnel: w4275 -> [w4290 w4310 w4365 w4368]
      tunnel: [enum16{"init", "MAIN", "Panel Close"}."MAIN" w4305 _ _] -> w4273
      frame "init" {
        n3299 = local read "Com Port 1"() -> (w4283:refnum<visa-resource-name>)
        n3300 = Bundle By Name(cluster=w4290, "Heave and Surge COM Port:"=w4283) -> (w4289:T18)
        n3301 = call "Instrument fgv uno.vi"("Enum"=T29."INIT", "error in (no error) 2"=w4293, "INPUT"=w4289) -> ("error"=w4291:errorcluster, "output"=w4287:T18)  [unwired: 6 in, 1 out]
        n3302 = case shown="Error" w4291 {
          selector: w4291 -> [w4295 _]
          tunnel: [w4295 w4299] -> w4288
          tunnel: w4287 -> [w4294 w4297]
          tunnel: [w4294 w4296] -> w4286
          frame No Error {
          }
          frame Error {
            n3303 = call "Instrument fgv uno.vi"("Enum"=T29."ERROR INIT", "INPUT"=w4297) -> ("error"=w4300:errorcluster, "output"=w4296:T18)  [unwired: 7 in, 1 out]
            n3304 = call <vilib>:"Clear Errors.vi"("error in (no error)"=w4300) -> ("error out"=w4299:errorcluster)  [unwired: 5 in, 1 out]
          }
        }
        n3305 = local read "LastCom Humidity"() -> (w4282:string)
        n3306 = Unbundle By Name(w4286) -> ("Heave COM Status 2"=→"COM Status":bool, "Error Heave"=→"Error":errorcluster)  [unwired: 1 out]
        n3307 = Bundle By Name(cluster=w4286, "LastCom"=w4282) -> (w4285:T18)
      }
      frame "MAIN" {
        n3308 = Unbundle By Name(w4310) -> ("Com Port 2"=w4317:refnum<visa-resource-name>)
        n3309 = local read "Com Port 1"() -> (w4304:refnum<visa-resource-name>)
        n3310 = local write "Com Port 5"(w4317) -> ()
        n3311 = Bundle By Name(cluster=w4310, "Heave and Surge COM Port:"=w4304) -> (w4309:T18)
        n3312 = Equal?(x=w4317, y=w4304) -> (x = y?=w4316:bool)
        n3313 = case shown="True" w4316 {
          tunnel: [w4321 w4338] -> w4315
          tunnel: w4311 -> [w4322 w4344]
          tunnel: w4309 -> [w4320 w4342]
          tunnel: [w4319 w4337] -> w4313
          frame False {
            n3314 = call <vilib>:"Clear Errors.vi"("error in (no error)"=w4322) -> ("error out"=w4318:errorcluster)  [unwired: 5 in, 1 out]
            n3315 = call "Instrument fgv uno.vi"("Enum"=T29."ERROR INIT", "error in (no error) 2"=w4318, "INPUT"=w4320) -> ("error"=w4324:errorcluster, "output"=w4319:T18)  [unwired: 6 in, 1 out]
            n3316 = call <vilib>:"Clear Errors.vi"("error in (no error)"=w4324) -> ("error out"=w4321:errorcluster)  [unwired: 5 in, 1 out]
          }
          frame True {
            n3317 = call "Instrument fgv uno.vi"("Enum"=T29."READ", "error in (no error) 2"=w4344, "INPUT"=w4342) -> ("error"=w4343:errorcluster, "output"=w4335:T18)  [unwired: 6 in, 1 out]
            n3318 = Bundle By Name(cluster=w4335, "String 36"="WRITE HUMIDITY") -> (w4334:T18)
            n3319 = case shown="True" "Write" {
              selector: "Write" -> [_ w4364]
              tunnel: w4343 -> [w4357 w4363]
              tunnel: [w4357 w4362] -> w4332
              tunnel: w4334 -> [w4356 w4359]
              tunnel: [w4356 w4358] -> w4331
              frame False {
              }
              frame True {
                n3320 = Not(x=w4364) -> (.not. x?=w4360:bool)
                n3321 = local write "Write"(w4360) -> ()
                n3322 = call "Instrument fgv uno.vi"("Enum"=T29."MANUAL WRITE", "error in (no error) 2"=w4363, "INPUT"=w4359) -> ("error"=w4362:errorcluster, "output"=w4358:T18)  [unwired: 6 in, 1 out]
              }
            }
            n3323 = Array Size(array="WriteHumidity") -> (size(s)=w4329:i32)
            n3324 = Greater Than 0?(x=w4329) -> (x > 0?=w4328:bool)
            n3325 = call "Instrument fgv uno.vi"("Enum"=T29."WRITE", "error in (no error) 2"=w4332, "WriteCC1"="WriteHumidity", "INPUT"=w4331) -> ("error"=w4340:errorcluster, "WriteCC1 2"=w4330:string[], "output"=w4339:T18)  [unwired: 5 in]
            n3326 = case shown="True" w4328 {
              tunnel: w4330 -> [_ w4346]
              frame False {
              }
              frame True {
                n3327 = local write "WriteHumidity"(w4346) -> ()
              }
            }
            n3328 = case shown="No Error" w4340 {
              selector: w4340 -> [w4347 w4350]
              tunnel: w4339 -> [w4348 w4355]
              tunnel: [w4348 w4354] -> w4337
              tunnel: [w4347 w4352] -> w4338
              frame No Error {
              }
              frame Error {
                n3329 = call <vilib>:"Clear Errors.vi"("error in (no error)"=w4350) -> ("error out"=w4349:errorcluster)  [unwired: 5 in, 1 out]
                n3330 = call "Instrument fgv uno.vi"("Enum"=T29."ERROR INIT", "error in (no error) 2"=w4349, "INPUT"=w4355) -> ("error"=w4353:errorcluster, "output"=w4354:T18)  [unwired: 6 in, 1 out]
                n3331 = call <vilib>:"Clear Errors.vi"("error in (no error)"=w4353) -> ("error out"=w4352:errorcluster)  [unwired: 5 in, 1 out]
              }
            }
            n3332 = Unbundle By Name(w4337) -> ("LastCom"=→"LastCom Humidity":string, "Read Heave and Surge"=→"Read HUMIDITY":string)
          }
        }
        n3333 = Unbundle By Name(w4313) -> ("Heave COM Status 2"=w4314:bool, "Error Heave"=w4301:errorcluster, "Bytes at Heave Port"=→"Bytes at Humidity Port  2":dbl)  [unwired: 1 out]
        n3334 = Unbundle By Name(w4301) -> ("status"=→"Humidity Port":bool)
        n3335 = Not(x=w4314) -> (.not. x?=w4302:bool)
        n3336 = local write "Error"(w4301) -> ()
        n3337 = local read "Quit"() -> (w4306:bool)
        n3338 = local write "COM Status"(w4302) -> ()
        n3339 = Select(t=enum16{"init", "MAIN", "Panel Close"}."Panel Close", s=w4306, f=enum16{"init", "MAIN", "Panel Close"}."MAIN") -> (s? t:f=w4305:enum16{"init", "MAIN", "Panel Close"})
      }
      frame "Panel Close" {
      }
      frame Default {
      }
    }
  }
  n3340 = while {
    shift-right: [w4375] -> _
    shift-left: _ -> [w4376]
    shift-right: [w4373] -> _
    shift-left: T18 {"Read Heave and Surge"="", "Bytes at Heave Port"=0.0, "Heave and Surge COM Port:"="COM9", "Com Port 2"="COM7", "Residual Due"="", "Heave COM Status 2"=TRUE, "Heave COM Status"=TRUE, "Port 2"=TRUE, "Sway PPR"=6400.0, "Surge PPR"=6400.0, "Heave PPR"=6400.0, "Sway Pitch"=2.0, "Surge Pitch"=3.0, "Heave Pitch"=4.0, "Sway Pulses/mm"=320.0, "Surge Pulses/mm"=1600.0, "Heave Pulses/mm"=1600.0, "inner loop"=0.0, "Read Heave and Surge 2"="", "String 36"="", "Write S"=FALSE, "WriteCC1"=[""], "Heave COM Loop"=0, "LastCom"="", "EXIT"=FALSE, "Error Heave"={"status"=TRUE, "code"=-1073807343, "source"=""}} -> [w4372]
    shift-right: [w4370] -> _
    shift-left: enum16{"init", "MAIN", "Panel Close"}."init" -> [w4371]
    stop <- w4374 stop-if-true
    # "UNO CODE LOGIC"
    n3341 = case shown="\"MAIN\"" w4371 {
      tunnel: w4376 -> [w4390 w4408 w4465 w4467]
      tunnel: [w4384 w4413 w4465 w4467] -> w4375
      tunnel: [_ _ TRUE _] -> w4374
      tunnel: [w4380 w4411 w4463 w4466] -> w4373
      tunnel: w4372 -> [w4387 w4407 w4463 w4466]
      tunnel: [enum16{"init", "MAIN", "Panel Close"}."MAIN" w4401 _ _] -> w4370
      frame "init" {
        n3342 = Bundle By Name(cluster=w4387, "Heave and Surge COM Port:"="C3 :") -> (w4386:T18)
        n3343 = call "Instrument fgv.vi"("Enum"=T29."INIT", "error in (no error) 2"=w4390, "INPUT"=w4386) -> ("error"=w4388:errorcluster, "output"=w4383:T18)  [unwired: 6 in, 1 out]
        n3344 = case shown="Error" w4388 {
          selector: w4388 -> [w4392 _]
          tunnel: [w4392 w4396] -> w4384
          tunnel: w4383 -> [w4391 w4394]
          tunnel: [w4391 w4393] -> w4381
          frame No Error {
          }
          frame Error {
            n3345 = call "Instrument fgv.vi"("Enum"=T29."ERROR INIT", "INPUT"=w4394) -> ("error"=w4397:errorcluster, "output"=w4393:T18)  [unwired: 7 in, 1 out]
            n3346 = call <vilib>:"Clear Errors.vi"("error in (no error)"=w4397) -> ("error out"=w4396:errorcluster)  [unwired: 5 in, 1 out]
          }
        }
        n3347 = local read "LastCom UNO"() -> (w4378:string)
        n3348 = Unbundle By Name(w4381) -> ("Heave COM Status 2"=→"Instrument Status":bool, "Error Heave"=→"Error  2":errorcluster)  [unwired: 1 out]
        n3349 = Bundle By Name(cluster=w4381, "LastCom"=w4378) -> (w4380:T18)
      }
      frame "MAIN" {
        n3350 = Unbundle By Name(w4407) -> ("Com Port 2"=w4415:refnum<visa-resource-name>)
        n3351 = local write "Com Port 4"(w4415) -> ()
        n3352 = local read "C3 :"() -> (w4405:refnum<visa-resource-name>)
        n3353 = Bundle By Name(cluster=w4407, "Heave and Surge COM Port:"=w4405) -> (w4406:T18)
        n3354 = Equal?(x=w4415, y=w4405) -> (x = y?=w4414:bool)
        n3355 = case shown="True" w4414 {
          tunnel: [w4419 w4436] -> w4413
          tunnel: w4408 -> [w4420 w4442]
          tunnel: w4406 -> [w4418 w4440]
          tunnel: [w4417 w4435] -> w4411
          frame False {
            n3356 = call <vilib>:"Clear Errors.vi"("error in (no error)"=w4420) -> ("error out"=w4416:errorcluster)  [unwired: 5 in, 1 out]
            n3357 = call "Instrument fgv.vi"("Enum"=T29."ERROR INIT", "error in (no error) 2"=w4416, "INPUT"=w4418) -> ("error"=w4422:errorcluster, "output"=w4417:T18)  [unwired: 6 in, 1 out]
            n3358 = call <vilib>:"Clear Errors.vi"("error in (no error)"=w4422) -> ("error out"=w4419:errorcluster)  [unwired: 5 in, 1 out]
          }
          frame True {
            n3359 = call "Instrument fgv.vi"("Enum"=T29."READ", "error in (no error) 2"=w4442, "INPUT"=w4440) -> ("error"=w4441:errorcluster, "output"=w4433:T18)  [unwired: 6 in, 1 out]
            n3360 = Bundle By Name(cluster=w4433, "String 36"="WRITE UNO") -> (w4432:T18)
            n3361 = case shown="True" "Write S" {
              selector: "Write S" -> [_ w4462]
              tunnel: w4441 -> [w4455 w4461]
              tunnel: [w4455 w4460] -> w4430
